vi "Override Equalization.vi"(0 "acq in":refnum<class "niUSRP Rx DSP v2 FPGA.lvclass">, 5 "equalization with registers":refnum<class "Equalization with Registers (IQ 18-bit).lvclass">) -> (4 "acq out":refnum<class "niUSRP Rx DSP v2 FPGA.lvclass">)   [LabVIEW 2025, in "niUSRP Rx DSP v2 FPGA.lvclass"]
uses:
  niUSRP Rx DSP v2 FPGA.lvclass
  <instrlib>/_niInstr/DSP Control/Common/v2/FPGA/Equalization/IQ 18-bit with Regs/Equalization with Registers (IQ 18-bit).lvclass
  C:/Program Files/NI/LVAddons/niidl/1/instr.lib/_niInstr/DSP Control/Interface/v1/FPGA/Equalization/IQ 18-bit/Equalization Interface (IQ 18-bit).lvclass
  <instrlib>/_niInstr/DSP Control/Interface/v1/FPGA/Equalization/IQ 18-bit/Equalization Interface (IQ 18-bit).lvclass
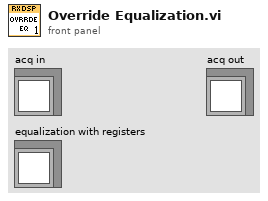
[diagram p1: front panel]
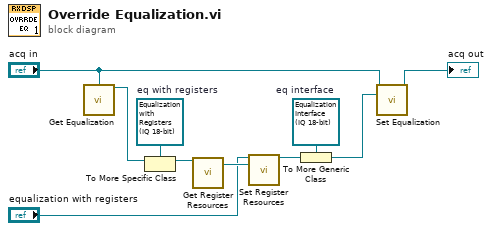
[diagram p0: block diagram]
diagram:
  w5 = refnum<class "Equalization with Registers (IQ 18-bit).lvclass"> refnum  # eq with registers
  w7 = refnum<class "Equalization Interface (IQ 18-bit).lvclass"> refnum  # eq interface
  n1 = call-dynamic "Get Equalization.vi"("acq in"="acq in") -> ("equalization"=w1:refnum<class "Equalization Interface (IQ 18-bit).lvclass">)  [unwired: 14 in]
  n2 = To More Specific Class(target class=w5, reference=w1) -> (specific class reference=w10:refnum<class "Equalization with Registers (IQ 18-bit).lvclass">)  [unwired: 1 in, 1 out]
  n3 = call <instrlib>:"Get Register Resources.vi"("equalization in"=w10) -> ("equalization regs"=w6:refnum<class "Equalization Registers.lvclass">)  [unwired: 13 in, 1 out]
  n4 = call <instrlib>:"Set Register Resources.vi"("equalization in"="equalization with registers", "equalization regs"=w6) -> ("equalization out"=w9:refnum<class "Equalization with Registers (IQ 18-bit).lvclass">)  [unwired: 13 in]
  n5 = To More Generic Class(target class=w7, reference=w9) -> (generic class reference=w8:refnum<class "Equalization Interface (IQ 18-bit).lvclass">)
  n6 = call-dynamic "Set Equalization.vi"("acq in"="acq in", "equalization"=w8) -> ("acq out"=→"acq out":refnum<class "niUSRP Rx DSP v2 FPGA.lvclass">)  [unwired: 13 in]
